vi "Volt to I16.vi"(1 "Voltage In":dbl) -> (0 "I16 Voltage Out":i16)   [LabVIEW 2014]
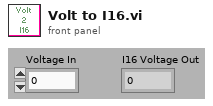
[diagram p1: front panel]
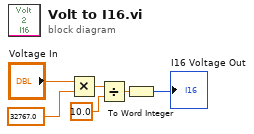
[diagram p0: block diagram]
diagram:
  n1 = Multiply(x="Voltage In", y=32767.0) -> (x*y=w6:dbl)
  n2 = Divide(x=w6, y=10.0) -> (x/y=w5:dbl)
  n3 = To Word Integer(number=w5) -> (16bit integer=→"I16 Voltage Out":i16)
